vi "ForceTorqueSensor.vi"() -> ()   [LabVIEW 2019]
uses:
  <vilib>/Platform/TimedLoop/XDataNode/timing_clust.ctl
  <vilib>/Platform/TimedLoop/XDataNode/nitl_modes.ctl
  <vilib>/Platform/TimedLoop/XDataNode/wakeup.ctl
  <vilib>/Analysis/3filter.llb/Filter Passband Type.ctl
  <vilib>/Analysis/baseanly.llb/Real Dot Product.vi
  <vilib>/Utility/file.llb/Write Delimited Spreadsheet (DBL).vi
  <vilib>/platform/TimedLoop/XDataNode/XDataNode.xnode
  <vilib>/Analysis/NI_AALBase.lvlib
  <vilib>/Platform/TimedLoop/XDataNode/XDNodeRunTimeDep.lvlib
  <vilib>/ptbypt/NI_PtbyPt.lvlib
panel:
  out "Finished Late? [i-1]":bool
  out "Mx":dbl[](graph) caption="Mx ="
  in  "MxData":path
  out "error out 3":errorcluster
  out "Cdb_Mx":dbl[](array[numeric])
  in  "StartAcq":bool
  in  "FxData":path
  out "error out 2":errorcluster
  out "error out":errorcluster
  out "Cdb_Fx":dbl[](array[numeric])
  out "Fx":dbl[](graph) caption="Fx ="
  in  "Unbias":bool
  out "Bias Vector":dbl[](array[numeric])
  in  "Bias":bool
  out "Voltages":dbl[][](array[numeric])
  in  "Guage Data":path
  in  "stop":bool
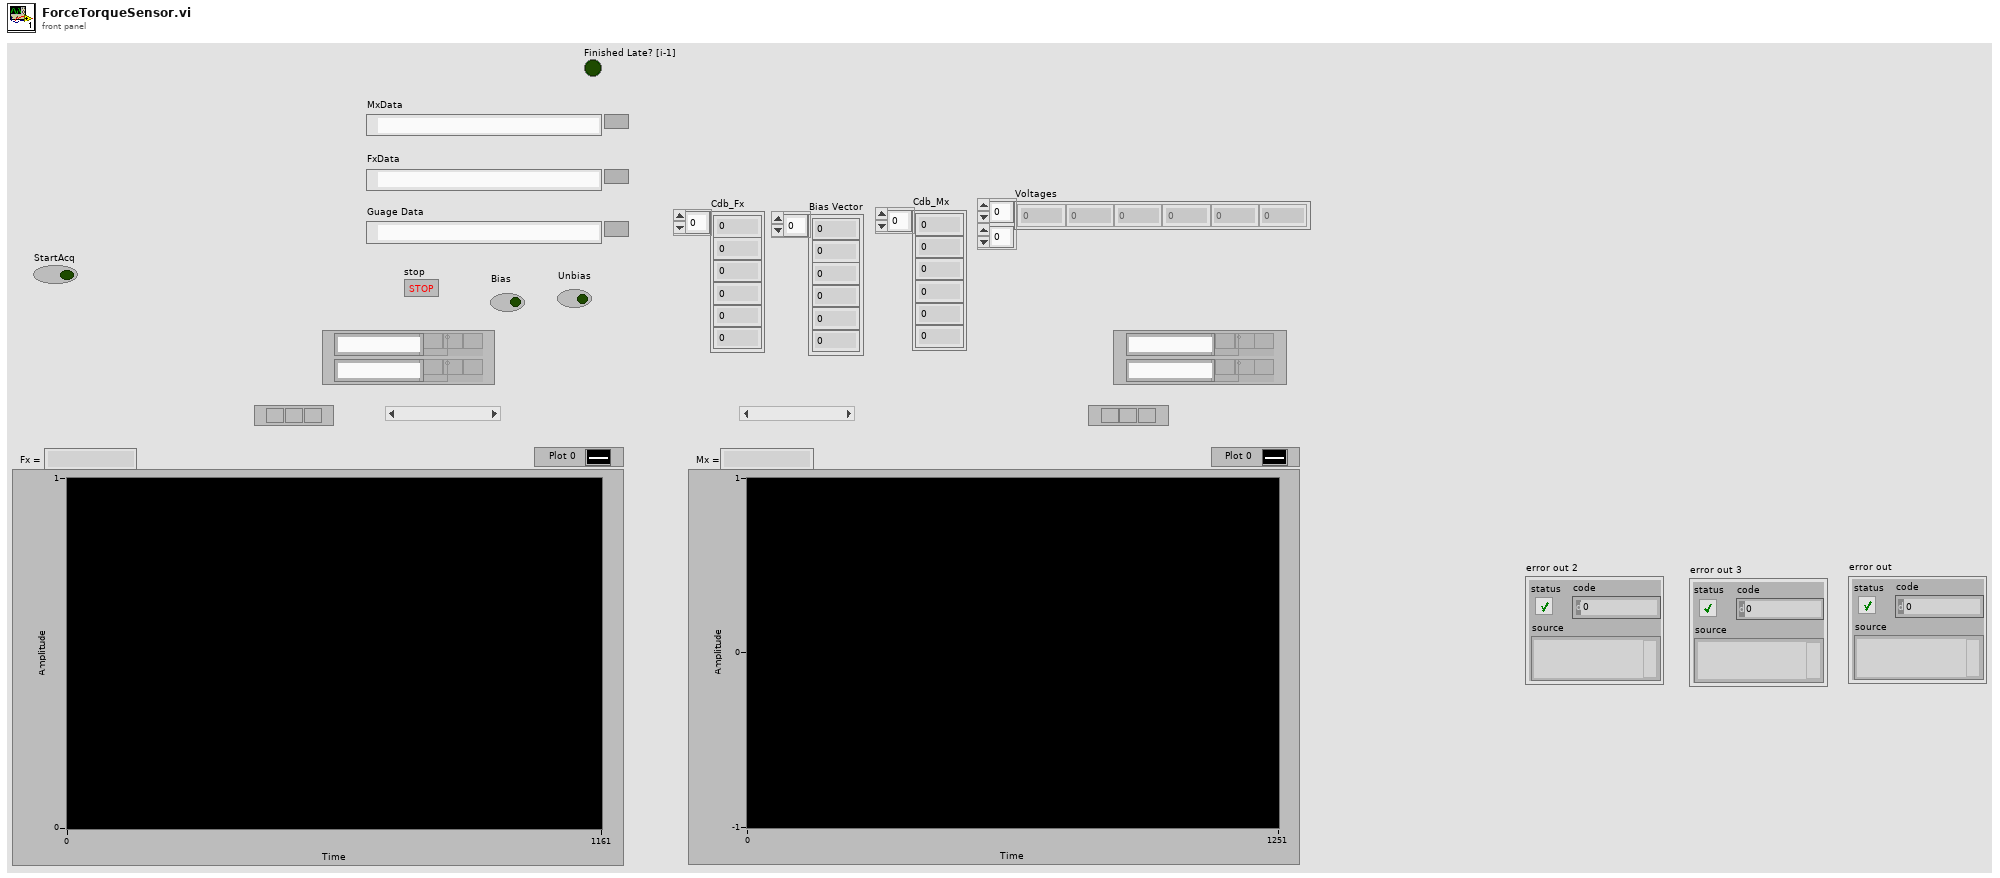
[diagram p1: front panel]
types:
  T1 = typedef "XDNodeRunTimeDep.lvlib/timing_clust.ctl" = cluster{"Expected End [f-1]":u64, "Actual End [f-1]":u64, "Finished Late? [f-1]":bool, "Expected End [i-1]":u64, "Actual End [i-1]":u64, "Finished Late? [i-1]":bool, "Expected Start [i]":u64, "Actual Start [i]":u64, "Expected Start [f]":u64, "Actual Start [f]":u64, "Source Name":string, "Structure Name":string, "Period":i64, "Deadline":i64, "Offset":i64, "Start":i64, "Priority":i32, "Timeout":i32, "Mode":T2, "Wakeup Reason":T3, "Error":errorcluster, "Source Type":string, "Secondary Source Type":string, "Global End Time":u64, "Global Start Time":u64, "Frame Duration":u64, "Iteration Duration":u64, "Assigned CPU":i32, "I/O Scan Engine Mode":u32}
  T2 = typedef "XDNodeRunTimeDep.lvlib/nitl_modes.ctl" = enum32{"No Change", "Process missed periods, maintain original phase", "Discard missed periods, maintain original phase", "Process missed periods, ignore original phase", "Discard missed periods, ignore original phase"}
  T3 = typedef "XDNodeRunTimeDep.lvlib/wakeup.ctl" = enum32{"Normal", "Aborted", "Asynchronous wakeup", "Timing source error", "Timed loop error", "Timeout"}
  T4 = typedef "NI_AALBase.lvlib/Filter Passband Type.ctl" = enum32{"Lowpass", "Highpass", "Bandpass", "Bandstop"}
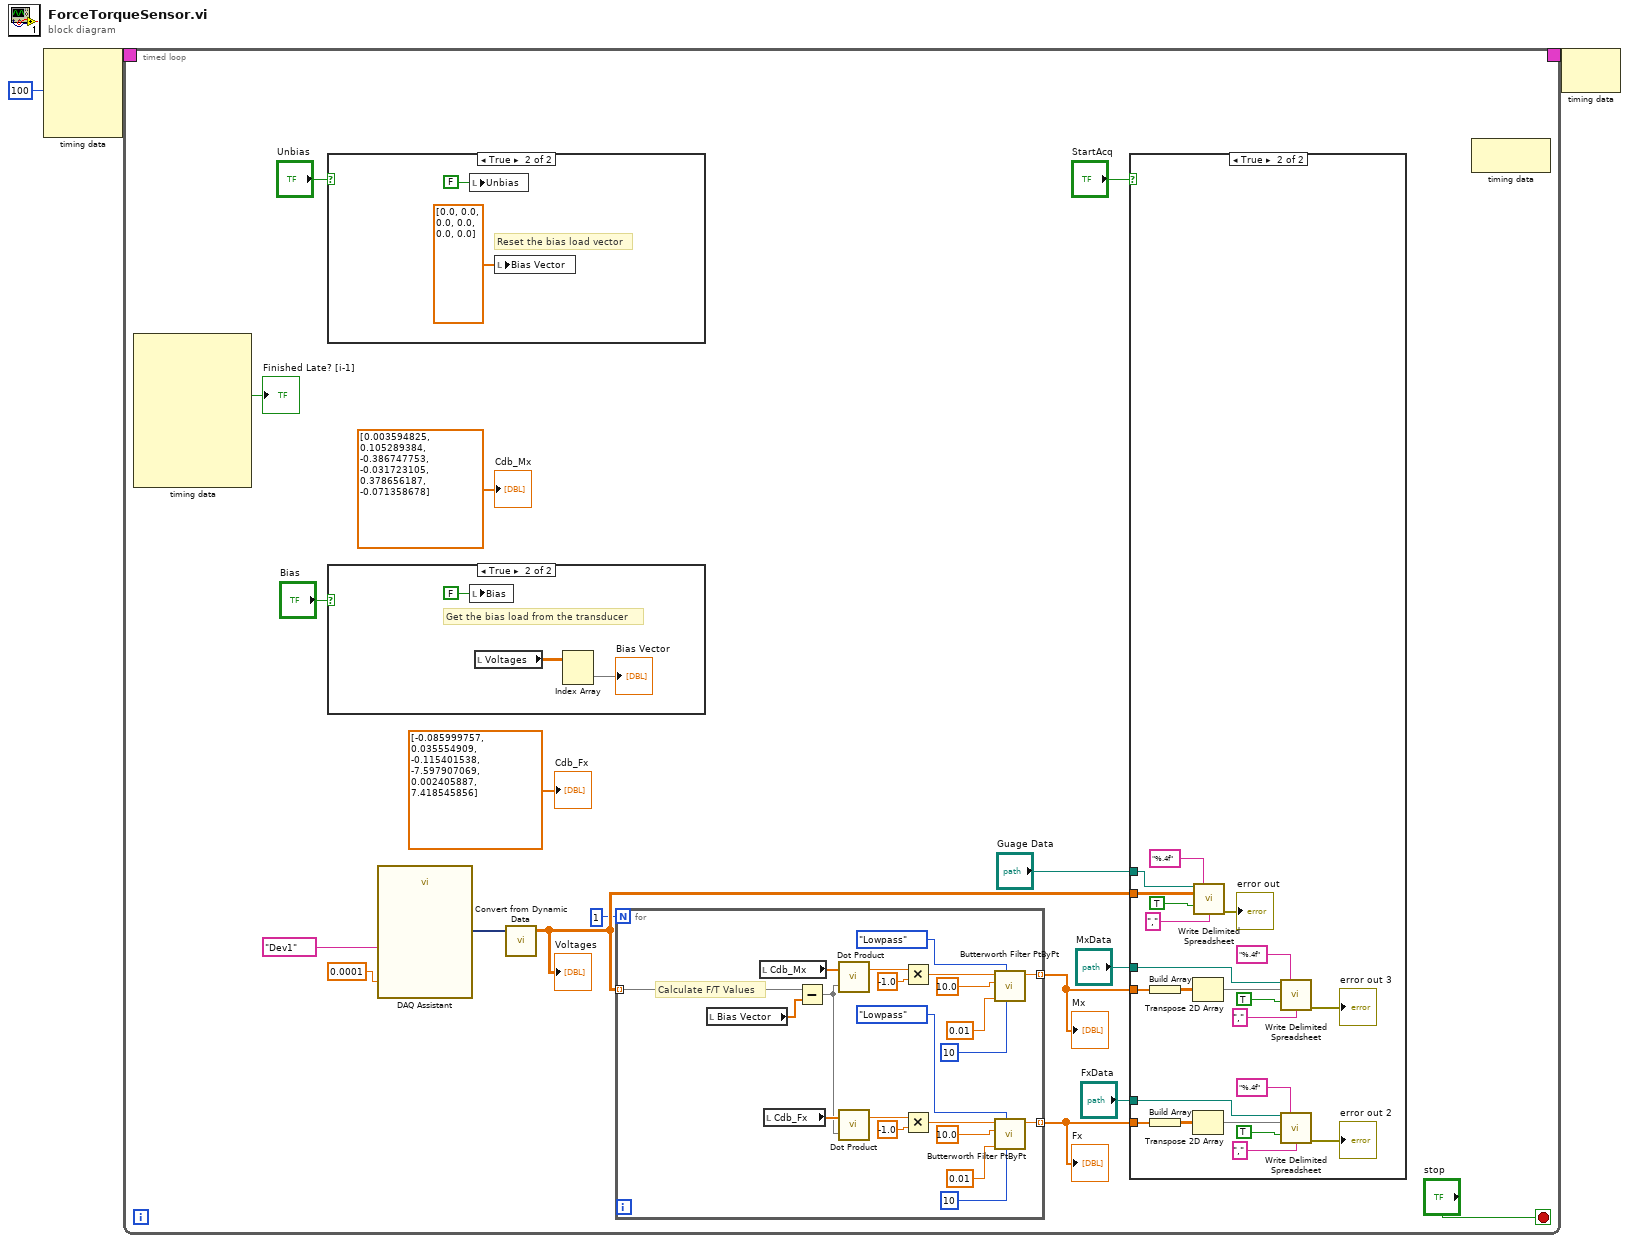
[diagram p0: block diagram]
diagram:
  n1 = node-c288(i64 100 ("Period")) -> (w3:T1)  [unwired: 3 in]
  n2 = timed-loop {
    timing: w3 -> [_]
    timing-out: [_] -> w2
    stop <- "stop" stop-if-true
    n3 = node-c288() -> (→"Finished Late? [i-1]":bool)  [unwired: 1 in, 8 out]
    n4 = case shown="True" "Unbias" {
      frame False {
      }
      frame True {
        # "Reset the bias load vector"
        n5 = local write "Unbias"(FALSE) -> ()
        n6 = local write "Bias Vector"(dbl[] [0.0, 0.0, 0.0, 0.0, 0.0, 0.0]) -> ()
      }
    }
    n7 = case shown="True" "Bias" {
      frame False {
      }
      frame True {
        # "Get the bias load from the transducer"
        n8 = local write "Bias"(FALSE) -> ()
        n9 = local read "Voltages"() -> (w49:dbl[][])
        n10 = Index Array(array=w49) -> (element=→"Bias Vector":dbl[])  [unwired: 2 in]
      }
    }
    n11 = call "DAQ Assistant"("timeout (s)"=0.0001, "device name"=tag "Dev1") -> ("data"=w12:dynamicdata)  [unwired: 15 in, 2 out]
    n12 = call "Convert from Dynamic Data"("Dynamic Data Type"=w12) -> ("Array"=w17:dbl[][])  [unwired: 3 in]
    "Voltages" <- w17
    n13 = for {
      N: 1 -> [_]
      tunnel: w17 -> [w46] mode=indexing
      tunnel: [w32] -> w11 mode=indexing
      tunnel: [w26] -> w6 mode=indexing
      # "Calculate F/T Values"
      n14 = local read "Bias Vector"() -> (w45:dbl[])
      n15 = local read "Cdb_Mx"() -> (w43:dbl[])
      n16 = local read "Cdb_Fx"() -> (w44:dbl[])
      n17 = Subtract(x=w46, y=w45) -> (x-y=w42:dbl[])
      n18 = call-poly <vilib>:"Dot Product.vi"("Y Vector"=w42, "X Vector"=w43) -> ("X * Y"=w41:dbl)  [unwired: 1 out]
      n19 = call-poly <vilib>:"Dot Product.vi"("Y Vector"=w42, "X Vector"=w44) -> ("X * Y"=w39:dbl)  [unwired: 1 out]
      n20 = Multiply(x=w41, y=-1.0) -> (x*y=w27:dbl)
      n21 = Multiply(x=w39, y=-1.0) -> (x*y=w33:dbl)
      n22 = call <vilib>:"Butterworth Filter PtByPt.vi"("order"=10, "filter type"=Filter_Passband_Type."Lowpass", "low cutoff freq: fl"=0.01, "sampling freq: fs"=10.0, "x"=w27) -> ("Filtered x"=w26:dbl)  [unwired: 4 in, 1 out]
      n23 = call <vilib>:"Butterworth Filter PtByPt.vi"("order"=10, "filter type"=Filter_Passband_Type."Lowpass", "low cutoff freq: fl"=0.01, "sampling freq: fs"=10.0, "x"=w33) -> ("Filtered x"=w32:dbl)  [unwired: 4 in, 1 out]
    }
    "Fx" <- w11
    "Mx" <- w6
    n24 = case shown="True" "StartAcq" {
      tunnel: "Guage Data" -> [_ w68]
      tunnel: w17 -> [_ w67]
      tunnel: w11 -> [_ w60]
      tunnel: "FxData" -> [_ w61]
      tunnel: "MxData" -> [_ w51]
      tunnel: w6 -> [_ w50]
      frame False {
      }
      frame True {
        n25 = Build Array(w50) -> (w53:dbl[][])
        n26 = Build Array(w60) -> (w59:dbl[][])
        n27 = Transpose 2D Array(2D array=w53) -> (transposed array=w52:dbl[][])
        n28 = Transpose 2D Array(2D array=w59) -> (transposed array=w58:dbl[][])
        n29 = call-poly <vilib>:"Write Delimited Spreadsheet.vi"("file path (dialog if empty)"=w68, "format (%.3f)"="%.4f", "2D data"=w67, "append to file? (new file:F)"=TRUE, "delimiter (\\t)"="," ("delimiter (\\t)")) -> ("error out"=→"error out":errorcluster)  [unwired: 9 in, 1 out]
        n30 = call-poly <vilib>:"Write Delimited Spreadsheet.vi"("file path (dialog if empty)"=w51, "format (%.3f)"="%.4f", "2D data"=w52, "append to file? (new file:F)"=TRUE, "delimiter (\\t)"="," ("delimiter (\\t)")) -> ("error out"=→"error out 3":errorcluster)  [unwired: 9 in, 1 out]
        n31 = call-poly <vilib>:"Write Delimited Spreadsheet.vi"("file path (dialog if empty)"=w61, "format (%.3f)"="%.4f", "2D data"=w58, "append to file? (new file:F)"=TRUE, "delimiter (\\t)"="," ("delimiter (\\t)")) -> ("error out"=→"error out 2":errorcluster)  [unwired: 9 in, 1 out]
      }
    }
    n32 = node-c288() -> ()  [unwired: 1 in, 1 out]
    "Cdb_Fx" <- dbl[] [-0.085999757, 0.035554909, -0.115401538, -7.597907069, 0.002405887, 7.418545856]
    "Cdb_Mx" <- dbl[] [0.003594825, 0.105289384, -0.386747753, -0.031723105, 0.378656187, -0.071358678] ("Cdb 2")
  }
  n33 = node-c288(w2) -> ()  [unwired: 1 out]
